vi "Set Up Terminal for Input Param.vi"(6 "ConPane Terminal Index":u32, 7 "CallLibrary Terminal Index":i32, 8 "error in (no error)":errorcluster, 9 "CalllLibrary Ref":refnum<vi>, 10 "VI Ref":refnum<vi>, 11 "Bool Writer in":refnum<class "Bool Writer.lvclass">) -> (0 "error out":errorcluster, 3 "Bool Writer out":refnum<class "Bool Writer.lvclass">)   [LabVIEW 2013, in "Bool Writer.lvclass"]
uses:
  Bool Writer.lvclass
  Abstract Param Writer/Abstract Param Writer.lvclass
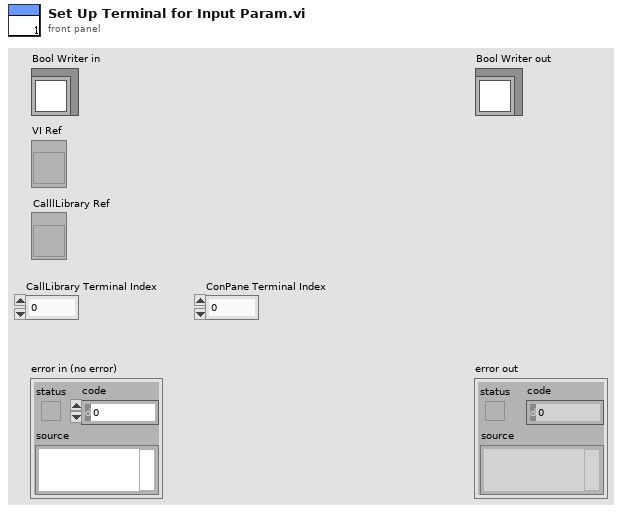
[diagram p1: front panel]
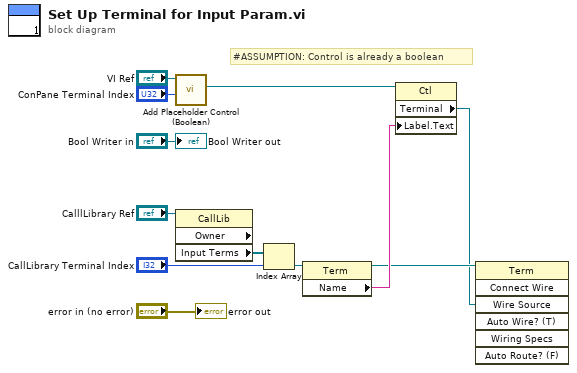
[diagram p0: block diagram]
diagram:
  # "#ASSUMPTION: Control is already a boolean"
  n1 = call "Add Placeholder Control (Boolean).vi"("ConPane Terminal Index"="ConPane Terminal Index", "VI Ref"="VI Ref") -> ("Control Ref"=w2:refnum<vi>)  [unwired: 9 in]
  n2 = property class="CallLib" props=["Owner", "Input Terms"](reference="CalllLibrary Ref") -> ("Input Terms"=w7:refnum<vi>[])  [unwired: 1 in, 3 out]
  n3 = Index Array(array=w7, index="CallLibrary Terminal Index") -> (element=w5:refnum<vi>)
  n4 = property class="Term"(reference=w5) -> (reference out=w3:refnum<vi>, "Name"=w4:string)  [unwired: 1 in, 1 out]
  n5 = property class="Ctl"(reference=w2, "Label.Text"=w4) -> ("Terminal"=w1:refnum<vi>)  [unwired: 1 in, 2 out]
  n6 = invoke class="Term" method="Connect Wire"(reference=w3, "Wire Source"=w1) -> ()  [unwired: 5 in, 7 out]
  "error out" <- "error in (no error)"
  "Bool Writer out" <- "Bool Writer in"
